vi "PathPlanner_Path_ConstTargetSpacing.vi"() -> (3 "TargetSpacing":dbl=0.2)   [LabVIEW 2019, in "PathPlanner24.lvlib"]
doc: "Get the number of points in this path\n\nInputs: \n - Path - cluster - path definition data structure\n\nOutputs:\n - NumPoints - integer - Number of points in the path"
uses:
  PathPlanner24.lvlib
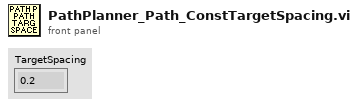
[diagram p1: front panel]
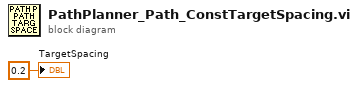
[diagram p0: block diagram]
diagram:
  "TargetSpacing" <- 0.2 ("TargetIncrement")
